vi "TestData_MySQL_Connect.vi"(8 "error in (no error)":errorcluster, 11 "ConnectionString":T1={"IP"="192.168.0.119", "Port"="3306", "DataBase"="uel_te", "User"="liguang", "Password"="delta343723"}) -> (0 "Error Out":errorcluster caption="错误输出", 3 "Connection Out":refnum<k7>)   [LabVIEW 2012, in "Lib_UEL.ATE.lvlib" / "Lib_TestData.lvlib"]
uses:
  Lib_TestData.lvlib
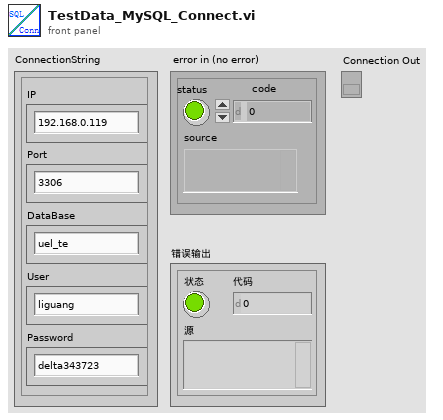
[diagram p1: front panel]
types:
  T1 = cluster{"IP":string, "Port":string, "DataBase":string, "User":string, "Password":string}
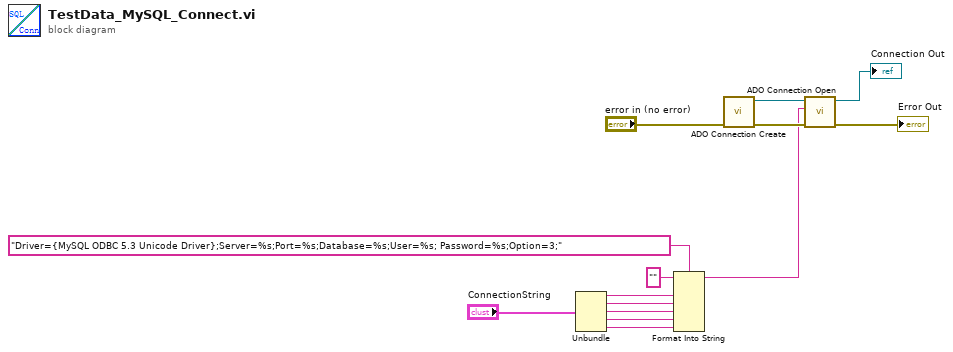
[diagram p0: block diagram]
diagram:
  n1 = Unbundle("ConnectionString") -> ("IP"=w11:string, "Port"=w10:string, "DataBase"=w9:string, "User"=w8:string, "Password"=w7:string)
  n2 = Format Into String(format string="Driver={MySQL ODBC 5.3 Unicode Driver};Server=%s;Port=%s;Database=%s;User=%s; Password=%s;Option=3;" ("格式字符串"), initial string="" ("初始字符串"), w11, w10, w9, w8, w7) -> (resulting string=w4:string)  [unwired: 1 in, 1 out]
  n3 = call <userlib>:"ADO Connection Create.vi"("error in (no error)"="error in (no error)") -> ("error out"=w6:errorcluster, "ADODB._Connection Out"=w3:refnum<k7>)  [unwired: 9 in]
  n4 = call <userlib>:"ADO Connection Open.vi"("error in (no error)"=w6, "ConnectionString"=w4, "ADODB._Connection In"=w3) -> ("error out"=→"Error Out":errorcluster, "ADODB._Connection Out"=→"Connection Out":refnum<k7>)  [unwired: 7 in]
